vi "main.vi"() -> ()   [LabVIEW 2012]
uses:
  <vilib>/Platform/TimedLoop/XDataNode/timing_clust.ctl
  <vilib>/Platform/TimedLoop/XDataNode/nitl_modes.ctl
  <vilib>/Platform/TimedLoop/XDataNode/wakeup.ctl
  <vilib>/Platform/TimedLoop/XDataNode/XDataNode.xnode
  <vilib>/Platform/TimedLoop/XDataNode/XDNodeRunTimeDep.lvlib
panel:
  out "K 2":i16
  out "able to shoot of Tank 2":bool
  in  "able to shoot of Tank 1":bool
  in  "stop":bool
  in  "Tank2AqFind":bool
  in  "Tank2AqAngle":dbl
  in  "Tank2":dbl[](array[numeric])=[-1.0, -1.0]
  in  "Tank1AqFind":bool
  in  "Tank1AqAngle":dbl
  in  "Tank1":dbl[](array[numeric])=[1.0, 1.0]
  in  "K":i16
  in  "dir2":dbl
  in  "dir1":dbl
  in  "Ball":dbl[](array[numeric])=[0.0, 0.0]
  # "1. 打开间谍卫星系统"
  # "2. 打开两个机器人的IPcamera"
  # "这里暂时手调"
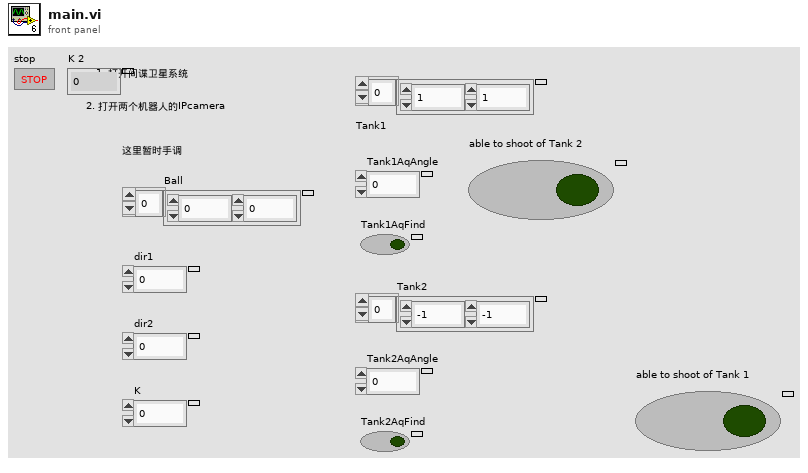
[diagram p1: front panel]
types:
  T1 = typedef "XDNodeRunTimeDep.lvlib/timing_clust.ctl" = cluster{"Expected End [f-1]":u64, "Actual End [f-1]":u64, "Finished Late? [f-1]":bool, "Expected End [i-1]":u64, "Actual End [i-1]":u64, "Finished Late? [i-1]":bool, "Expected Start [i]":u64, "Actual Start [i]":u64, "Expected Start [f]":u64, "Actual Start [f]":u64, "Source Name":string, "Structure Name":string, "Period":i64, "Deadline":i64, "Offset":i64, "Start":i64, "Priority":i32, "Timeout":i32, "Mode":T2, "Wakeup Reason":T3, "Error":errorcluster, "Source Type":string, "Secondary Source Type":string, "Global End Time":u64, "Global Start Time":u64, "Frame Duration":u64, "Iteration Duration":u64, "Assigned CPU":i32, "I/O Scan Engine Mode":u32}
  T2 = typedef "XDNodeRunTimeDep.lvlib/nitl_modes.ctl" = enum32{"No Change", "Process missed periods, maintain original phase", "Discard missed periods, maintain original phase", "Process missed periods, ignore original phase", "Discard missed periods, ignore original phase"}
  T3 = typedef "XDNodeRunTimeDep.lvlib/wakeup.ctl" = enum32{"Normal", "Aborted", "Asynchronous wakeup", "Timing source error", "Timed loop error", "Timeout"}
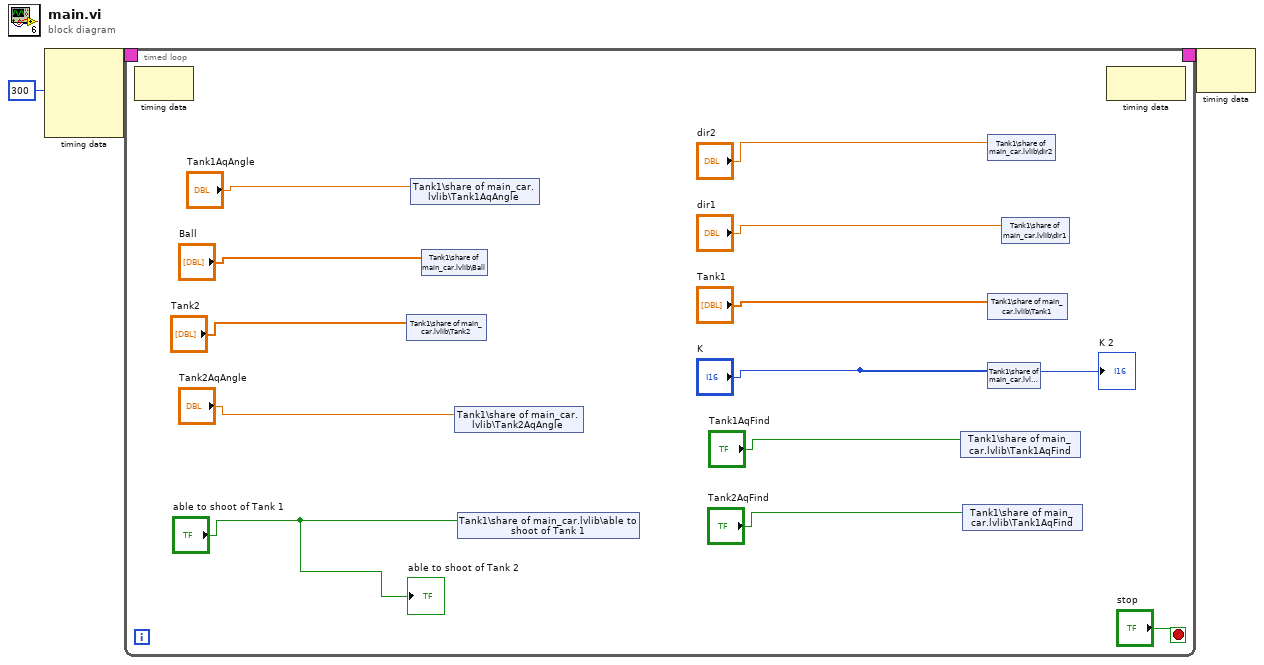
[diagram p0: block diagram]
diagram:
  n1 = node-c288(i64 300 ("Period")) -> (w3:T1)  [unwired: 3 in]
  n2 = timed-loop {
    timing: w3 -> [_]
    timing-out: [_] -> w2
    stop <- "stop" stop-if-true
    n3 = node-c288() -> ()  [unwired: 1 in, 1 out]
    n4 = shared-variable "Tank1\\share of main_car.lvlib\\Tank2"("Tank2") -> ()  [unwired: 1 in, 1 out]
    n5 = shared-variable "Tank1\\share of main_car.lvlib\\Tank1AqAngle"("Tank1AqAngle") -> ()  [unwired: 1 in, 1 out]
    n6 = shared-variable "Tank1\\share of main_car.lvlib\\Ball"("Ball") -> ()  [unwired: 1 in, 1 out]
    n7 = shared-variable "Tank1\\share of main_car.lvlib\\Tank2AqAngle"("Tank2AqAngle") -> ()  [unwired: 1 in, 1 out]
    n8 = shared-variable "Tank1\\share of main_car.lvlib\\able to shoot of Tank 1"("able to shoot of Tank 1") -> ()  [unwired: 1 in, 1 out]
    n9 = shared-variable "Tank1\\share of main_car.lvlib\\Tank1AqFind"("Tank1AqFind") -> ()  [unwired: 1 in, 1 out]
    n10 = shared-variable "Tank1\\share of main_car.lvlib\\Tank1AqFind"("Tank2AqFind") -> ()  [unwired: 1 in, 1 out]
    n11 = shared-variable "Tank1\\share of main_car.lvlib\\dir2"("dir2") -> ()  [unwired: 1 in, 1 out]
    n12 = shared-variable "Tank1\\share of main_car.lvlib\\Tank1"("Tank1") -> ()  [unwired: 1 in, 1 out]
    n13 = shared-variable "Tank1\\share of main_car.lvlib\\K"("K") -> ()  [unwired: 1 in, 1 out]
    n14 = shared-variable "Tank1\\share of main_car.lvlib\\dir1"("dir1") -> ()  [unwired: 1 in, 1 out]
    n15 = node-c288() -> ()  [unwired: 1 in, 1 out]
    "able to shoot of Tank 2" <- "able to shoot of Tank 1"
    "K 2" <- "K"
  }
  n16 = node-c288(w2) -> ()  [unwired: 1 out]
